vi "patternmatching.vi"() -> ()   [LabVIEW 2019]
panel:
  out "count":i16
  in  "Array":string[](array[string])
  out "Data size(s)":i32
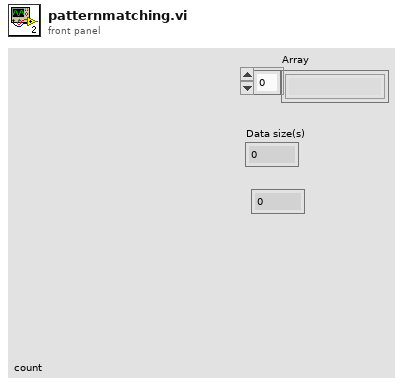
[diagram p1: front panel]
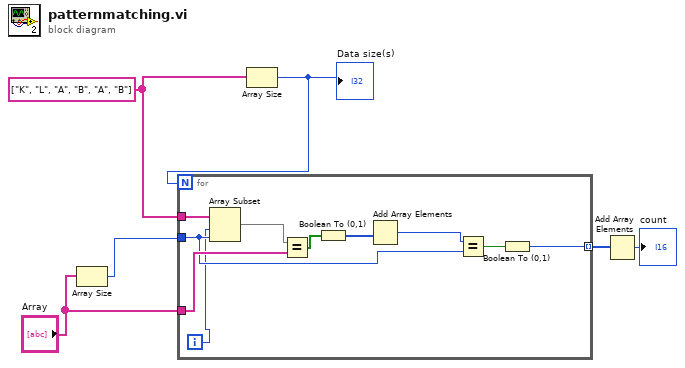
[diagram p0: block diagram]
diagram:
  w4 = string[] ["K", "L", "A", "B", "A", "B"]
  n1 = Array Size(array="Array") -> (size(s)=w3:i32)
  n2 = Array Size(array=w4) -> (size(s)=w6:i32)
  "Data size(s)" <- w6
  n3 = for {
    N: w6 -> [_]
    tunnel: "Array" -> [w16]
    tunnel: w4 -> [w15]
    tunnel: w3 -> [w13]
    tunnel: [w9] -> w2 mode=indexing
    i -> [w8]
    n4 = Array Subset(array=w15, index=w8, length=w13) -> (w14:string[])
    n5 = Equal?(x=w14, y=w16) -> (x = y?=w11:bool[])
    n6 = Boolean To (0,1)(Boolean=w11) -> (0, 1=w10:i16[])
    n7 = Add Array Elements(numeric array=w10) -> (sum=w12:i16)
    n8 = Equal?(x=w12, y=w13) -> (x = y?=w7:bool)
    n9 = Boolean To (0,1)(Boolean=w7) -> (0, 1=w9:i16)
  }
  n10 = Add Array Elements(numeric array=w2) -> (sum=→"count":i16)
